vi "Core Action.vi"(8 "error in (no error)":errorcluster, 10 "SECS-II Class":refnum<class "SECS-II Class.lvclass">, 11 "22-Host Sends Information to Equipment in":refnum<class "22-Host Sends Information to Equipment.lvclass">) -> (0 "error out":errorcluster, 2 "SECS-II Class Out":refnum<class "SECS-II Class.lvclass">, 3 "22-Host Sends Information to Equipment out":refnum<class "22-Host Sends Information to Equipment.lvclass">)   [LabVIEW 2020, in "SECS Scenarios.lvlib" / "22-Host Sends Information to Equipment.lvclass"]
uses:
  22-Host Sends Information to Equipment.lvclass
  D:/Dropbox/SECS/SECS_GEM v1.1.0/Com/SECS Scenarios/Scenarios Class/Scenarios Class.lvclass
  SECS Communication/SECS-II Class/SECS-II Class.lvclass
  SECS Communication/S10 Message Class/S10 Message Class.lvclass
  D:/Dropbox/SECS/SECS_GEM v1.1.0/Com/SECS Communication/SECS-II Class/SECS-II Class.lvclass
  Scenarios Class/Reply State.ctl
  Scenarios Class/Scenarios Class.lvclass/Scenarios Class.ctl
  Scenarios Class/Write Reply State.vi
  Scenarios Class/Read HSMS Class.vi
  SECS Communication/HSMS Class/HSMS Class.lvclass
  Scenarios Class/Scenarios Class.lvclass
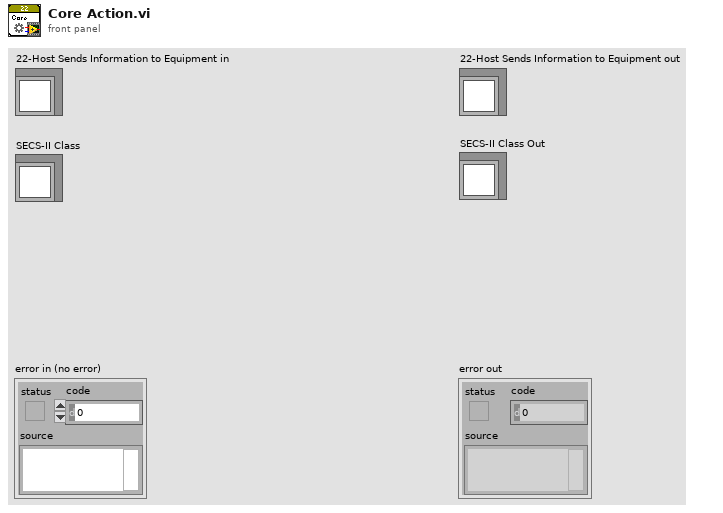
[diagram p1: front panel]
types:
  T1 = typedef "SECS Communication.lvlib/S10 Message Class.lvclass/S10F3.ctl" = cluster{"TID":u8, "TEXT":string}
  T2 = typedef "SECS Scenarios.lvlib/Scenarios Class.lvclass/Reply State.ctl" = enum16{"OK", "Illegal Data", "Unknown Stream", "Unknown Function", "Off-Line", "T3 Timeout", "Inner-Timeout"}
  T3 = typedef "SECS Communication.lvlib/S10 Message Class.lvclass/S10F4.ctl" = enum8{"accepted for display", "message will not be displayed", "terminal not available"}
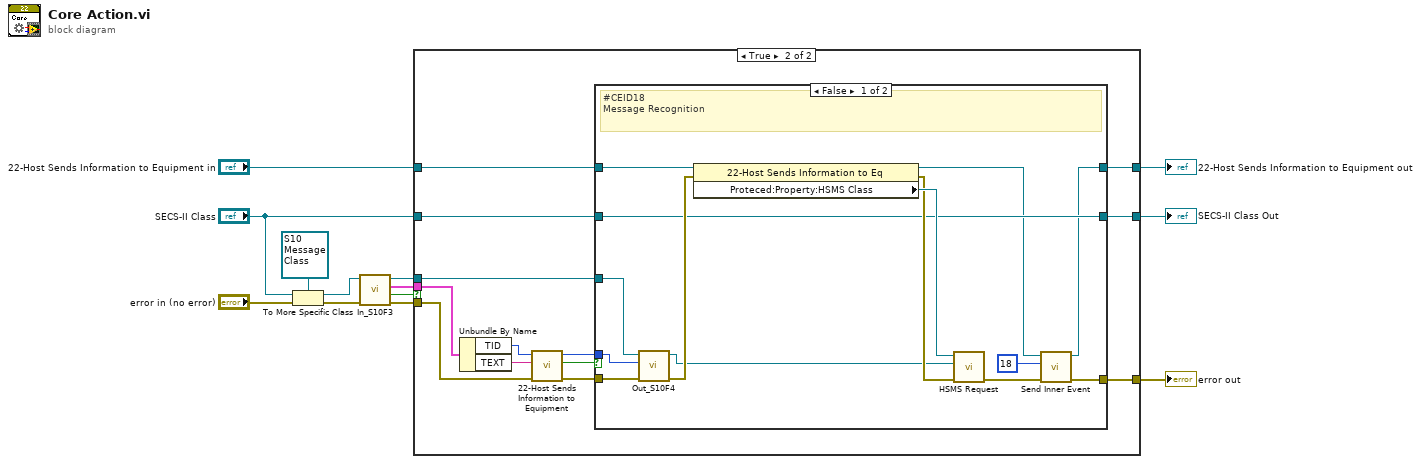
[diagram p0: block diagram]
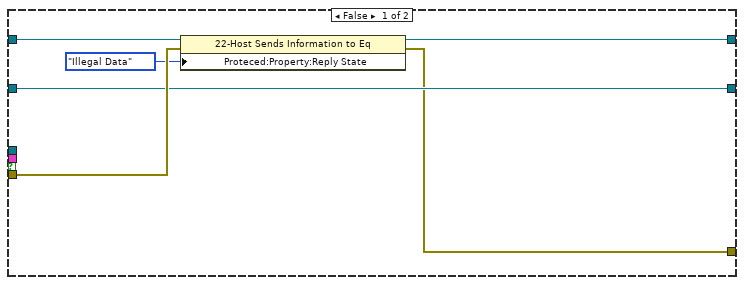
[diagram p2: hidden frame]
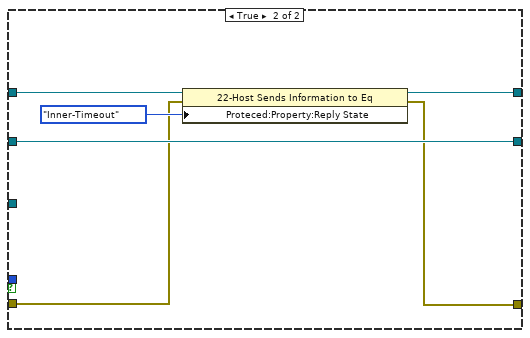
[diagram p3: hidden frame]
diagram:
  n1 = To More Specific Class(target class=refnum<class "S10 Message Class.lvclass"> refnum ("SECS Communication.lvlib:S10 Message Class.lvclass"), reference="SECS-II Class", error in="error in (no error)") -> (specific class reference=w12:refnum<class "S10 Message Class.lvclass">, error out=w13:errorcluster)
  n2 = call "In_S10F3.vi"("error in (no error)"=w13, "S10 Message Class in"=w12) -> ("error out"=w11:errorcluster, "OK?"=w1:bool, "S10F3"=w6:T1, "S10 Message Class out"=w10:refnum<class "S10 Message Class.lvclass">)  [unwired: 6 in]
  n3 = case shown="True" w1 {
    tunnel: w11 -> [w17 w32]
    tunnel: w10 -> [_ w31]
    tunnel: "22-Host Sends Information to Equipment in" -> [w19 w30]
    tunnel: w6 -> [_ w27]
    tunnel: [w14 w23] -> w5
    tunnel: [w18 w22] -> w4
    tunnel: "SECS-II Class" -> [w15 w21]
    tunnel: [w15 w20] -> w2
    frame False {
      n4 = property class="22-Host Sends Information to Eq"(reference=w19, error in=w17, "Proteced:Property:Reply State"=Reply_State."Illegal Data" ("Reply State")) -> (reference out=w18:refnum<class "22-Host Sends Information to Equipment.lvclass">, error out=w14:errorcluster)
    }
    frame True {
      n5 = Unbundle By Name(w27) -> ("TID"=w25:u8, "TEXT"=w26:string)
      n6 = call "22-Host Sends Information to Equipment.vi"("error in (no error)"=w32, "TEXT"=w26, "TID"=w25) -> ("error out"=w29:errorcluster, "Timeout?"=w28:bool, "S10F4"=w24:T3)  [unwired: 6 in]
      n7 = case shown="False" w28 {
        tunnel: w30 -> [w46 w50]
        tunnel: w31 -> [w39 _]
        tunnel: [w34 w47] -> w23
        tunnel: [w33 w48] -> w22
        tunnel: w29 -> [w43 w49]
        tunnel: w24 -> [w40 _]
        tunnel: w21 -> [w38 w52]
        tunnel: [w38 w52] -> w20
        frame False {
          # "#CEID18\nMessage Recognition"
          n8 = call "Out_S10F4.vi"("error in (no error)"=w43, "S10F4"=w40, "S10 Message Class in"=w39) -> ("error out"=w42:errorcluster, "S10 Message Class out"=w41:refnum<class "S10 Message Class.lvclass">)  [unwired: 7 in]
          n9 = property class="22-Host Sends Information to Eq"(reference=w46, error in=w42) -> (reference out=w35:refnum<class "22-Host Sends Information to Equipment.lvclass">, error out=w44:errorcluster, "Proteced:Property:HSMS Class"=w45:refnum<class "HSMS Class.lvclass">)
          n10 = call "HSMS Request.vi"("error in (no error)"=w44, "SECS-II Class In"=w41, "HSMS Class in"=w45) -> ("error out"=w37:errorcluster)  [unwired: 7 in, 1 out]
          n11 = call "Send Inner Event.vi"("error in (no error)"=w37, "CEID"=u32 18, "Scenarios Class in"=w35) -> ("error out"=w34:errorcluster, "Scenarios Class out"=w33:refnum<class "22-Host Sends Information to Equipment.lvclass">)  [unwired: 7 in]
        }
        frame True {
          n12 = property class="22-Host Sends Information to Eq"(reference=w50, error in=w49, "Proteced:Property:Reply State"=Reply_State."Inner-Timeout" ("Reply State")) -> (reference out=w48:refnum<class "22-Host Sends Information to Equipment.lvclass">, error out=w47:errorcluster)
        }
      }
    }
  }
  "error out" <- w5
  "22-Host Sends Information to Equipment out" <- w4
  "SECS-II Class Out" <- w2
